vi "Get Plot at Mouse Click [AAC].vi"(8 "error in (no error)":errorcluster, 10 "Mouse Click Coordinates":T1, 11 "XYGraph Ref":T2) -> (0 "error out":errorcluster, 1 "Click is in Legend?":bool, 2 "Plot at Coordinates":i32, 3 "XYGraph Ref":T2, 4 "Plot Name":string, 5 "Graph Caption":string, 6 "Found?":bool)   [LabVIEW 2019]
uses:
  XY Graph Refnum.ctl
  <vilib>/Utility/miscctls.llb/LVPoint32TypeDef.ctl
  XY Graph Add-Ons.lvlib
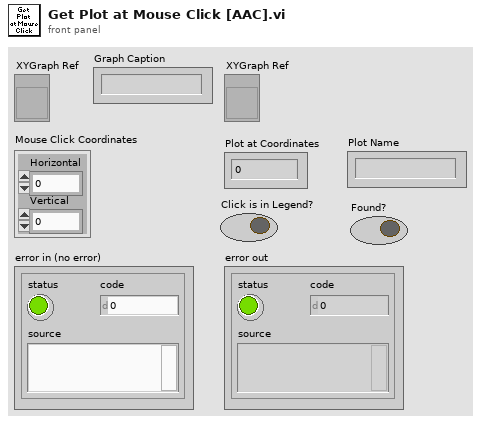
[diagram p1: front panel]
types:
  T1 = typedef "LVPoint32TypeDef.ctl" = cluster{"Horizontal":i32, "Vertical":i32}
  T2 = typedef "XY Graph Add-Ons.lvlib/XY Graph Refnum.ctl" = refnum<vi>
  T3 = typedef "LVPositionTypeDef.ctl" = cluster{"Left":i32, "Top":i32}
  T4 = typedef "LVBoundsTypeDef.ctl" = cluster{"Width":u32, "Height":u32}
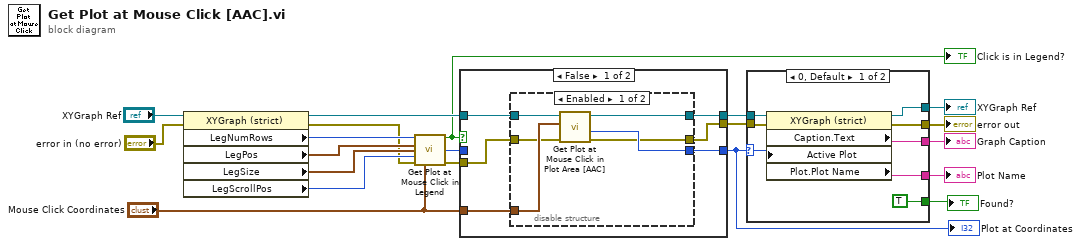
[diagram p0: block diagram]
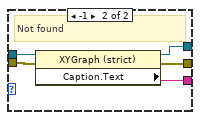
[diagram p2: hidden frame]
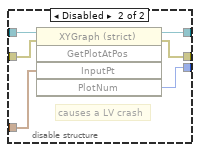
[diagram p3: hidden frame]
diagram:
  n1 = property class="XYGraph (strict)"(reference="XYGraph Ref", error in="error in (no error)") -> (reference out=w17:T2, error out=w9:errorcluster, "LegNumRows"=w18:u32, "LegPos"=w14:T3, "LegSize"=w13:T4, "LegScrollPos"=w12:u32)
  n2 = call "Get Plot at Mouse Click in Legend.vi"("LegNumRows"=w18, "Legend:Position"=w14, "Legend:Size"=w13, "LegScrollPos"=w12, "Error In"=w9, "Mouse Click Coordinates"="Mouse Click Coordinates") -> ("Click is in Legend?"=w16:bool, "Plot Index"=w10:i32, "Error Out"=w8:errorcluster)  [unwired: 7 in]
  "Click is in Legend?" <- w16
  n3 = case shown="False" w16 {
    tunnel: w17 -> [w23 w41]
    tunnel: [w26 w41] -> w19
    tunnel: w10 -> [_ w40]
    tunnel: [w25 w40] -> w3
    tunnel: "Mouse Click Coordinates" -> [w24 _]
    tunnel: w8 -> [w22 w39]
    tunnel: [w21 w39] -> w5
    frame False {
      n4 = disable-structure shown="Enabled" {
        disable-tunnel: [w32 w37] -> w26
        disable-tunnel: [w31 w33] -> w25
        disable-tunnel: w24 -> [w30 w35]
        disable-tunnel: w23 -> [w29 w38]
        disable-tunnel: w22 -> [w28 w36]
        disable-tunnel: [w27 w34] -> w21
        frame Enabled {
          n5 = call "Get Plot at Mouse Click in Plot Area [AAC].vi"("error in (no error)"=w28, "Mouse Click Coordinates (defaut: last plot)"=w30, "XYGraph Ref"=w29) -> ("error out"=w27:errorcluster, "Plot Index"=w31:i32, "XYGraph Ref"=w32:T2)  [unwired: 6 in]
        }
        frame Disabled {
          # "causes a LV crash"
          n6 = invoke class="XYGraph (strict)" method="GetPlotAtPos"(reference=w38, error in=w36, "InputPt"=w35) -> (reference out=w37:T2, error out=w34:errorcluster, "PlotNum"=w33:i32)  [unwired: 2 in, 2 out]
        }
      }
    }
    frame True {
      # "In the Legend Region"
    }
  }
  "Plot at Coordinates" <- w3
  n7 = case shown="0, Default" w3 {
    selector: w3 -> [w44 _]
    tunnel: w19 -> [w49 w54]
    tunnel: [w48 w50] -> w7
    tunnel: [w47 w52] -> w6
    tunnel: w5 -> [w46 w53]
    tunnel: [w45 w51] -> w4
    tunnel: [w43 _] -> w2
    tunnel: [TRUE ("Found?") _] -> w1
    frame 0, Default {
      n8 = property class="XYGraph (strict)"(reference=w49, error in=w46, "Active Plot"=w44) -> (reference out=w48:T2, error out=w45:errorcluster, "Caption.Text"=w47:string, "Plot.Plot Name"=w43:string)
    }
    frame -1 {
      # "Not found"
      n9 = property class="XYGraph (strict)"(reference=w54, error in=w53) -> (reference out=w50:T2, error out=w51:errorcluster, "Caption.Text"=w52:string)
    }
  }
  "error out" <- w4
  "XYGraph Ref" <- w7
  "Graph Caption" <- w6
  "Plot Name" <- w2
  "Found?" <- w1
